vi "predict_time_domain_python.vi"(1 "Module Path":path, 2 "SHG-Matrix":dbl[][](array[numeric]), 3 "error in (no error)":errorcluster, 4 "Header":string) -> (0 "error out":errorcluster)   [LabVIEW 2019]
panel:
  # "Description:\nUses SHG-Matrix and Header to predict the corresponding time domain signal using python"
  # "Inputs:"
  # "Outputs:"
  # "Array that contains the SHG-Matrix Header in the following order:\n1. Number of delay values\n2. Number of wavelength values\n3. \\delta_tau in [fs]\n4. \\delta_lambda in [nm]\n5. Center Wavelength [nm]"
  # "2D Array containing the SHG-Matrix"
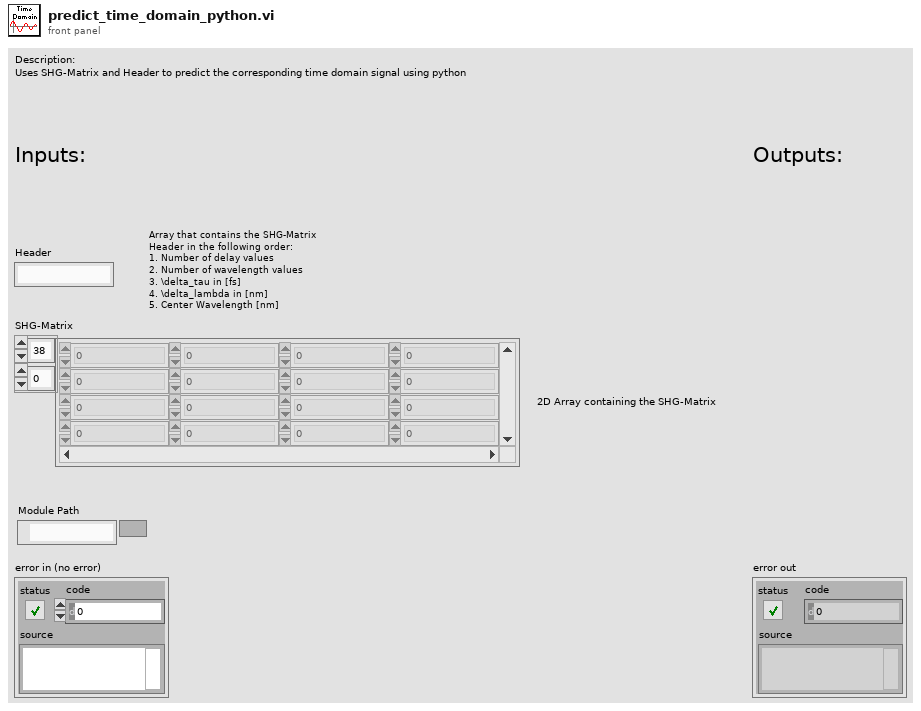
[diagram p1: front panel]
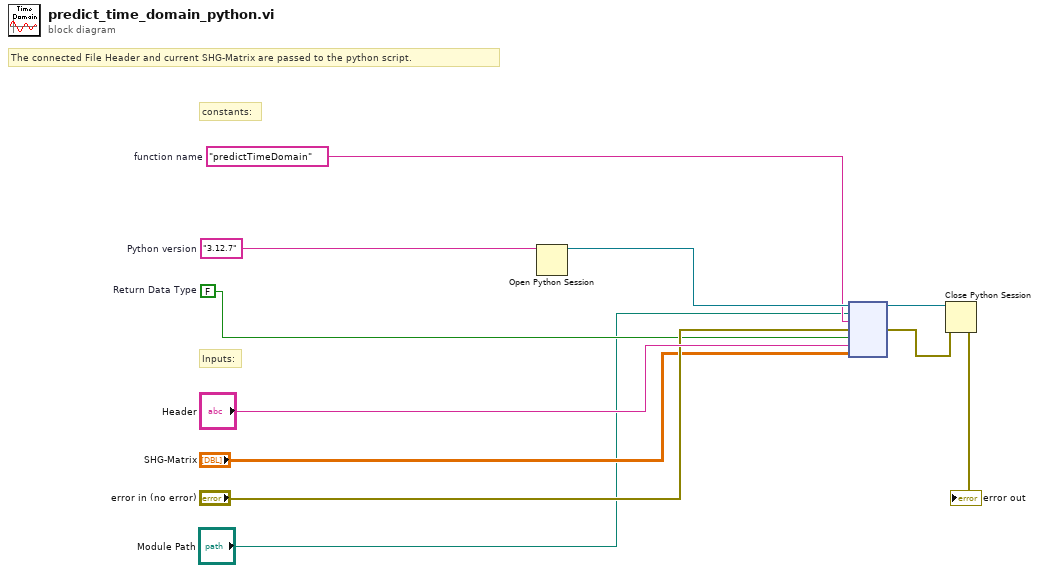
[diagram p0: block diagram]
diagram:
  w3 = FALSE  # Return Data Type
  w4 = "predictTimeDomain"  # function name
  w2 = "3.12.7"  # Python version
  # "constants:"
  # "Inputs:"
  # "The connected File Header and current SHG-Matrix are passed to the python script."
  n1 = Open Python Session(python version=w2) -> (session out=w5:refnum<k35>)  [unwired: 2 in, 1 out]
  n2 = node(w5, "Module Path", w4, "error in (no error)", w3, "Header", "SHG-Matrix") -> (w10:refnum<k35>, w8:errorcluster)  [unwired: 3 in, 2 out]
  n3 = Close Python Session(session in=w10, error in=w8) -> (11:→"error out":errorcluster)
